vi "MacroRules_FGV.vi"(7 "MacroRules_FGV_Commands":T1, 8 "Error In":errorcluster, 11 "Command Name IN":string) -> (0 "Error Out":errorcluster, 2 "Flags":string[](array[string]), 3 "Parameters":string[][](array[string]), 4 "FlagsTable":string[][](array[string]), 5 "ParametersTable":string[][](array[string]))   [LabVIEW 2017]
doc: "SciScan 1.2 160622\nThis VI reads the paramaters and flags relevant to the Macro Generator and stores itin an FGV. The User can query a Macro Command to get:\na. 2 D array containing all function arguments and their type\nb. 1D array containing a list of all flags it must listen to"
uses:
  MacroRules_FGV_Commands.ctl
  <vilib>/Utility/file.llb/Read From Spreadsheet File (string).vi
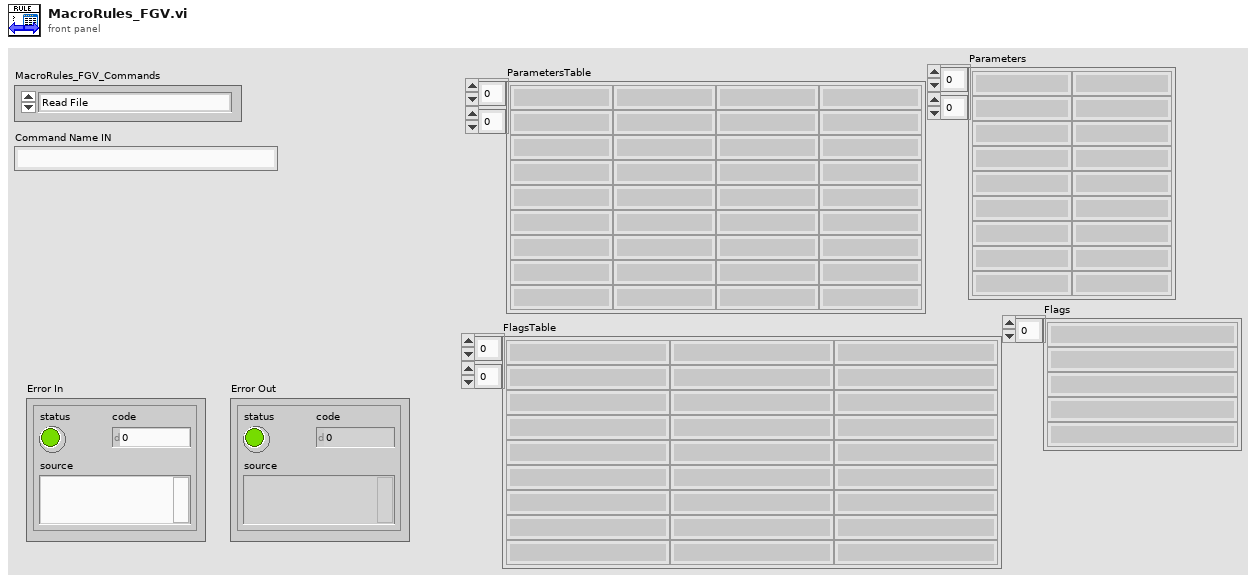
[diagram p1: front panel]
types:
  T1 = typedef "MacroRules_FGV_Commands.ctl" = enum16{"Read File", "Get All", "Get Param and Flags"}
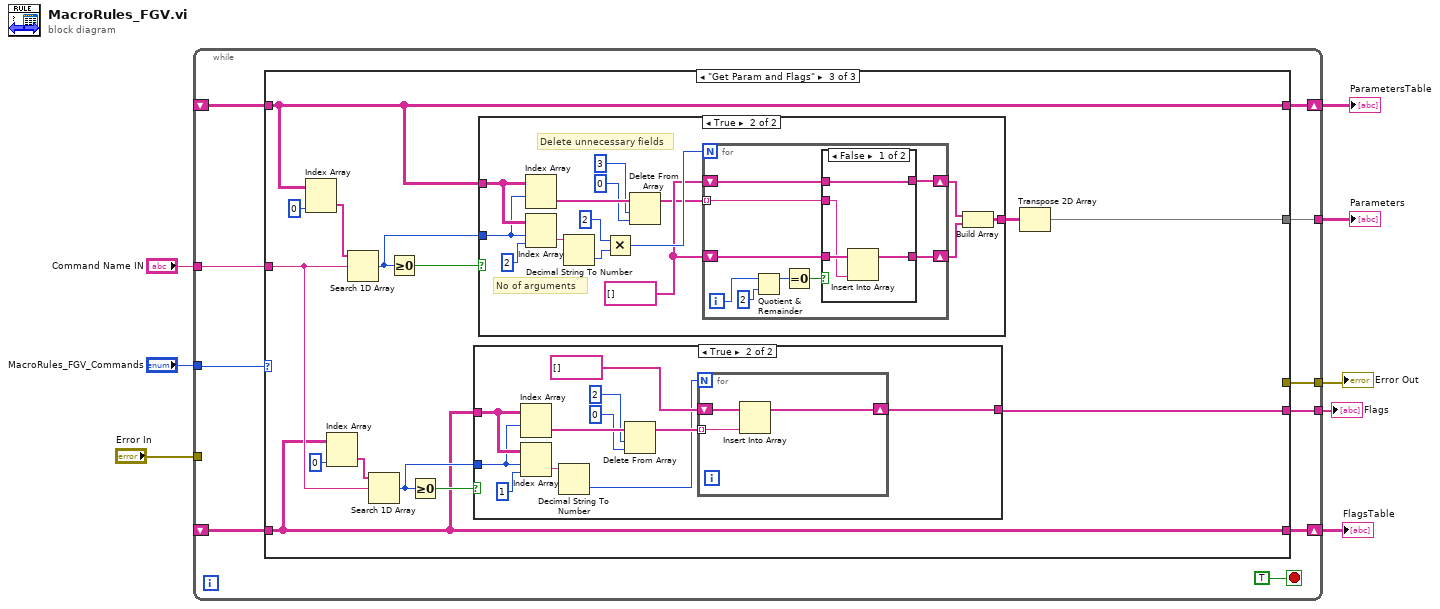
[diagram p0: block diagram]
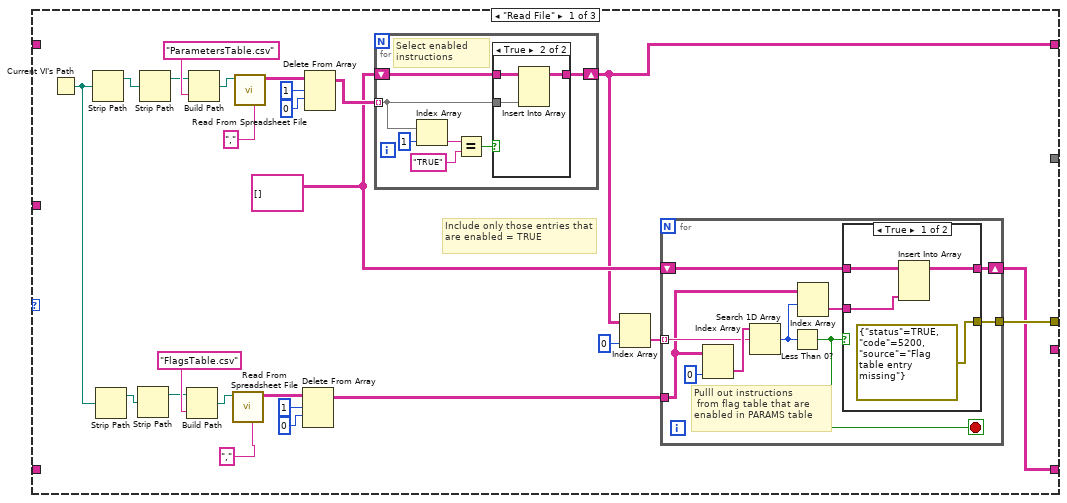
[diagram p2: hidden frame]
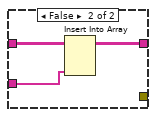
[diagram p3: hidden frame]
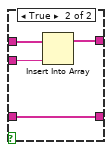
[diagram p8: hidden frame]
diagram:
  n1 = while {
    tunnel: "MacroRules_FGV_Commands" -> [w17]
    shift-right: [w16] -> w7
    shift-left: _ -> [w15]
    shift-right: [w14] -> w6
    shift-left: _ -> [w13]
    tunnel: "Command Name IN" -> [w12]
    tunnel: [w11] -> w4
    tunnel: [w10] -> w3
    tunnel: "Error In" -> [_]
    tunnel: [w9] -> w1
    stop <- TRUE stop-if-true
    n2 = case shown="\"Get Param and Flags\"" w17 {
      tunnel: [w19 w73 w83] -> w16
      tunnel: w15 -> [_ w73 w83]
      tunnel: [w20 w72 w75] -> w14
      tunnel: w13 -> [_ w72 w75]
      tunnel: w12 -> [_ _ w78]
      tunnel: [_ _ w81] -> w11
      tunnel: [_ _ w74] -> w10
      tunnel: [w22 _ _] -> w9
      frame "Read File" {
        w21 = string[][] [] ("array w/ subset deleted")
        # "Include only those entries that are enabled = TRUE"
        n3 = Current VI's Path() -> (path=w31:path)
        n4 = Strip Path(path=w31) -> (stripped path=w30:path)  [unwired: 1 out]
        n5 = Strip Path(path=w31) -> (stripped path=w29:path)  [unwired: 1 out]
        n6 = Strip Path(path=w29) -> (stripped path=w28:path)  [unwired: 1 out]
        n7 = Strip Path(path=w30) -> (stripped path=w27:path)  [unwired: 1 out]
        n8 = Build Path(base path=w28, name or relative path="FlagsTable.csv") -> (appended path=w36:path)
        n9 = Build Path(base path=w27, name or relative path="ParametersTable.csv") -> (appended path=w39:path)
        n10 = call-poly <vilib>:"Read From Spreadsheet File.vi"("delimiter (\\t)"="," ("delimiter (\\t)"), "file path (dialog if empty)"=w36) -> ("all rows"=w33:string[][])  [unwired: 5 in, 4 out]
        n11 = call-poly <vilib>:"Read From Spreadsheet File.vi"("delimiter (\\t)"="," ("delimiter (\\t)"), "file path (dialog if empty)"=w39) -> ("all rows"=w42:string[][])  [unwired: 5 in, 4 out]
        n12 = Delete From Array(array=w33, length=1, index (row)=0) -> (array with subset deleted=w26:string[][])  [unwired: 1 in, 1 out]
        n13 = Delete From Array(array=w42, length=1, index (row)=0) -> (array with subset deleted=w25:string[][])  [unwired: 1 in, 1 out]
        n14 = for {
          tunnel: w25 -> [w62] mode=indexing
          shift-right: [w61] -> w19
          shift-left: w21 -> [w63]
          # "Select enabled instructions"
          n15 = Index Array(array=w62, index=1 ("disabled index (col)")) -> (element=w66:string)
          n16 = Equal?(x=w66, y="TRUE") -> (x = y?=w64:bool)
          n17 = case shown="True" w64 {
            tunnel: w63 -> [w68 w71]
            tunnel: w62 -> [_ w70]
            tunnel: [w68 w69] -> w61
            frame False {
            }
            frame True {
              n18 = Insert Into Array(array=w71, new element=w70) -> (w69:string[][])  [unwired: 2 in]
            }
          }
        }
        n19 = Index Array(array=w19, index (col)=0 ("disabled index (col)")) -> (element=w23:string[])  [unwired: 1 in]
        n20 = for {
          tunnel: w23 -> [w51] mode=indexing
          tunnel: w26 -> [w48]
          tunnel: [w49] -> w22
          shift-right: [w44] -> w20
          shift-left: w21 -> [w47]
          stop <- w50 stop-if-true
          # "Pulll out instructions\n from flag table that are enabled in PARAMS table"
          n21 = Index Array(array=w48, index (col)=0 ("disabled index (col)")) -> (element=w52:string[])  [unwired: 1 in]
          n22 = Search 1D Array(1D array=w52, element=w51) -> (index of element=w46:i32)  [unwired: 1 in]
          n23 = Less Than 0?(x=w46) -> (x < 0?=w50:bool)
          n24 = Index Array(array=w48, index (row)=w46) -> (element=w45:string[])  [unwired: 1 in]
          n25 = case shown="True" w50 {
            tunnel: [errorcluster {"status"=TRUE, "code"=5200, "source"="Flag table entry missing"} ("error constant") _] -> w49
            tunnel: w47 -> [w56 w60]
            tunnel: w45 -> [w55 w59]
            tunnel: [w54 w58] -> w44
            frame True {
              n26 = Insert Into Array(array=w56, new element=w55) -> (w54:string[][])  [unwired: 2 in]
            }
            frame False {
              n27 = Insert Into Array(array=w60, new element=w59) -> (w58:string[][])  [unwired: 2 in]
            }
          }
        }
      }
      frame "Get All", Default {
      }
      frame "Get Param and Flags" {
        n28 = Index Array(array=w83, index (col)=0 ("disabled index (col)")) -> (element=w86:string[])  [unwired: 1 in]
        n29 = Index Array(array=w75, index (col)=0 ("disabled index (col)")) -> (element=w80:string[])  [unwired: 1 in]
        n30 = Search 1D Array(1D array=w86, element=w78) -> (index of element=w84:i32)  [unwired: 1 in]
        n31 = Search 1D Array(1D array=w80, element=w78) -> (index of element=w76:i32)  [unwired: 1 in]
        n32 = Greater Or Equal To 0?(x=w84) -> (x >= 0?=w85:bool)
        n33 = Greater Or Equal To 0?(x=w76) -> (x >= 0?=w77:bool)
        n34 = case shown="True" w77 {
          tunnel: w75 -> [_ w96]
          tunnel: w76 -> [_ w95]
          tunnel: [_ w89] -> w74
          frame False {
          }
          frame True {
            n35 = Index Array(array=w96, index (row)=w95) -> (element=w93:string[])  [unwired: 1 in]
            n36 = Index Array(array=w96, index (row)=w95, index (col)=1 ("disabled index (col)")) -> (element=w97:string)
            n37 = Decimal String To Number(string=w97) -> (number=w88:i32)  [unwired: 2 in, 1 out]
            n38 = Delete From Array(array=w93, length=2, index=0) -> (array with subset deleted=w92:string[])  [unwired: 1 out]
            n39 = for {
              N: w88 -> [_]
              tunnel: w92 -> [w100] mode=indexing
              shift-right: [w99] -> w89
              shift-left: string[] [] -> [w101]
              n40 = Insert Into Array(array=w101, new element=w100) -> (w99:string[])  [unwired: 1 in]
            }
          }
        }
        n41 = case shown="True" w85 {
          tunnel: w83 -> [_ w111]
          tunnel: w84 -> [_ w110]
          tunnel: [_ w106] -> w82
          frame False {
          }
          frame True {
            w109 = string[] []
            # "Delete unnecessary fields"
            # "No of arguments"
            n42 = Index Array(array=w111, index (row)=w110) -> (element=w105:string[])  [unwired: 1 in]
            n43 = Index Array(array=w111, index (row)=w110, index (col)=2 ("disabled index (col)")) -> (element=w115:string)
            n44 = Decimal String To Number(string=w115) -> (number=w114:i32)  [unwired: 2 in, 1 out]
            n45 = Multiply(x=2, y=w114) -> (x*y=w112:i32)
            n46 = Delete From Array(array=w105, length=3, index=0) -> (array with subset deleted=w104:string[])  [unwired: 1 out]
            n47 = for {
              N: w112 -> [_]
              tunnel: w104 -> [w120] mode=indexing
              shift-right: [w117] -> w108
              shift-left: w109 -> [w121]
              shift-right: [w118] -> w107
              shift-left: w109 -> [w119]
              i -> [w125]
              n48 = Quotient & Remainder(x=w125, y=2) -> (x-y*floor(x/y)=w123:i32)  [unwired: 1 out]
              n49 = Equal To 0?(x=w123) -> (x = 0?=w122:bool)
              n50 = case shown="False" w122 {
                tunnel: w121 -> [w126 w133]
                tunnel: w120 -> [w128 w132]
                tunnel: w119 -> [w129 w131]
                tunnel: [w127 w131] -> w118
                tunnel: [w126 w130] -> w117
                frame False {
                  n51 = Insert Into Array(array=w129, new element=w128) -> (w127:string[])  [unwired: 1 in]
                }
                frame True {
                  n52 = Insert Into Array(array=w133, new element=w132) -> (w130:string[])  [unwired: 1 in]
                }
              }
            }
            n53 = Build Array(w108, w107) -> (w106:string[][])
          }
        }
        n54 = Transpose 2D Array(2D array=w82) -> (transposed array=w81:string[][])
      }
    }
  }
  "Error Out" <- w1
  "ParametersTable" <- w7
  "FlagsTable" <- w6
  "Parameters" <- w4
  "Flags" <- w3
